vi "Example_Single.vi"() -> ()   [LabVIEW 2015, in "LXM32_Modbus_Serial.lvlib"]
uses:
  LXM32_Modbus_Serial.lvlib
  statistic_indicator.ctl
  register_param.ctl
  <vilib>/Utility/sysdir.llb/System Directory Type.ctl
  <vilib>/Analysis/baseanly.llb/Mean (DBL).vi
  <vilib>/Utility/file.llb/Write Delimited Spreadsheet (string).vi
  <vilib>/Utility/file.llb/Write Delimited Spreadsheet (DBL).vi
  <vilib>/Analysis/NI_AALBase.lvlib
panel:
  in  "Test Name":string="Test"
  in  "Parameter":i32(ring)=3 items=["DC Bus [V]", "Motor Current[Arms]", "Motor Volt [V]", "Actual Torque [%]", "Actual Speed Rot. [rpm]", "Actual Speed Rot. Enc [rpm]", "Actual Velocity", "Actual Velocity of Enc.", "Actual Pos.", "Actual pos. of Enc"]
  in  "LXM Port":refnum<visa-resource-name>
  in  "Stop":bool
  in  "avg":T1={"value"=999.999, "desc"="DC BUS [V]"} caption="Average" {"value" format="%.3f"}
  in  "min":T1={"value"=999.999, "desc"="DC BUS [V]"} caption="Minimum" {"value" format="%.3f"}
  in  "max":T1={"value"=999.999, "desc"="DC BUS [V]"} caption="Maximum" {"value" format="%.3f"}
  in  "nowValue":T1={"value"=999.999, "desc"="DC BUS [V]"} caption="Now Value" {"value" format="%.3f"}
  out "chart":dbl[](graph) caption="Waveform Chart"
  # "LXM32 MODBUS SERIAL"
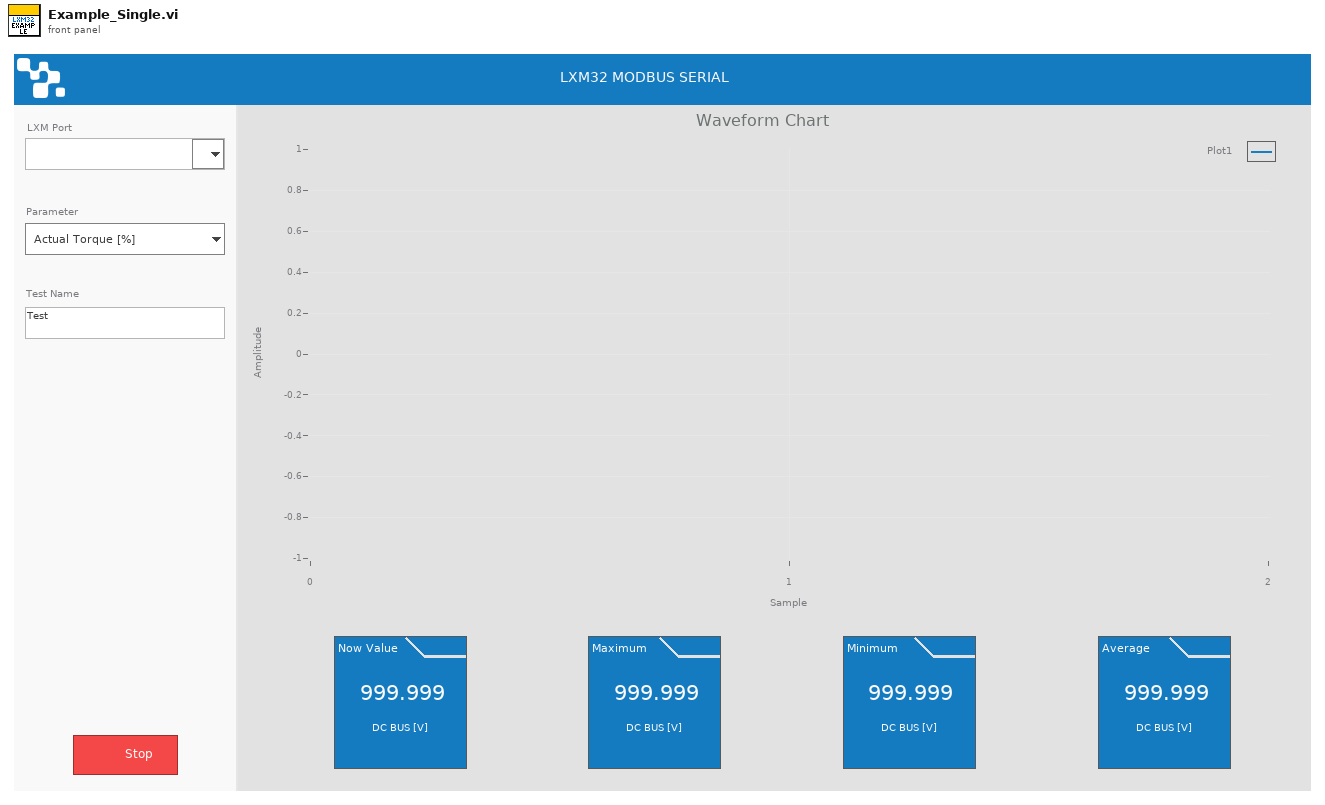
[diagram p1: front panel]
types:
  T1 = typedef "LXM32_Modbus_Serial.lvlib/statistic_indicator.ctl" = cluster{"value":dbl, "desc":string}
  T2 = typedef "System Directory Type.ctl" = i32
  T3 = typedef "LXM32_Modbus_Serial.lvlib/register_param.ctl" = cluster{"name":string, "address":u16, "divisor":dbl}
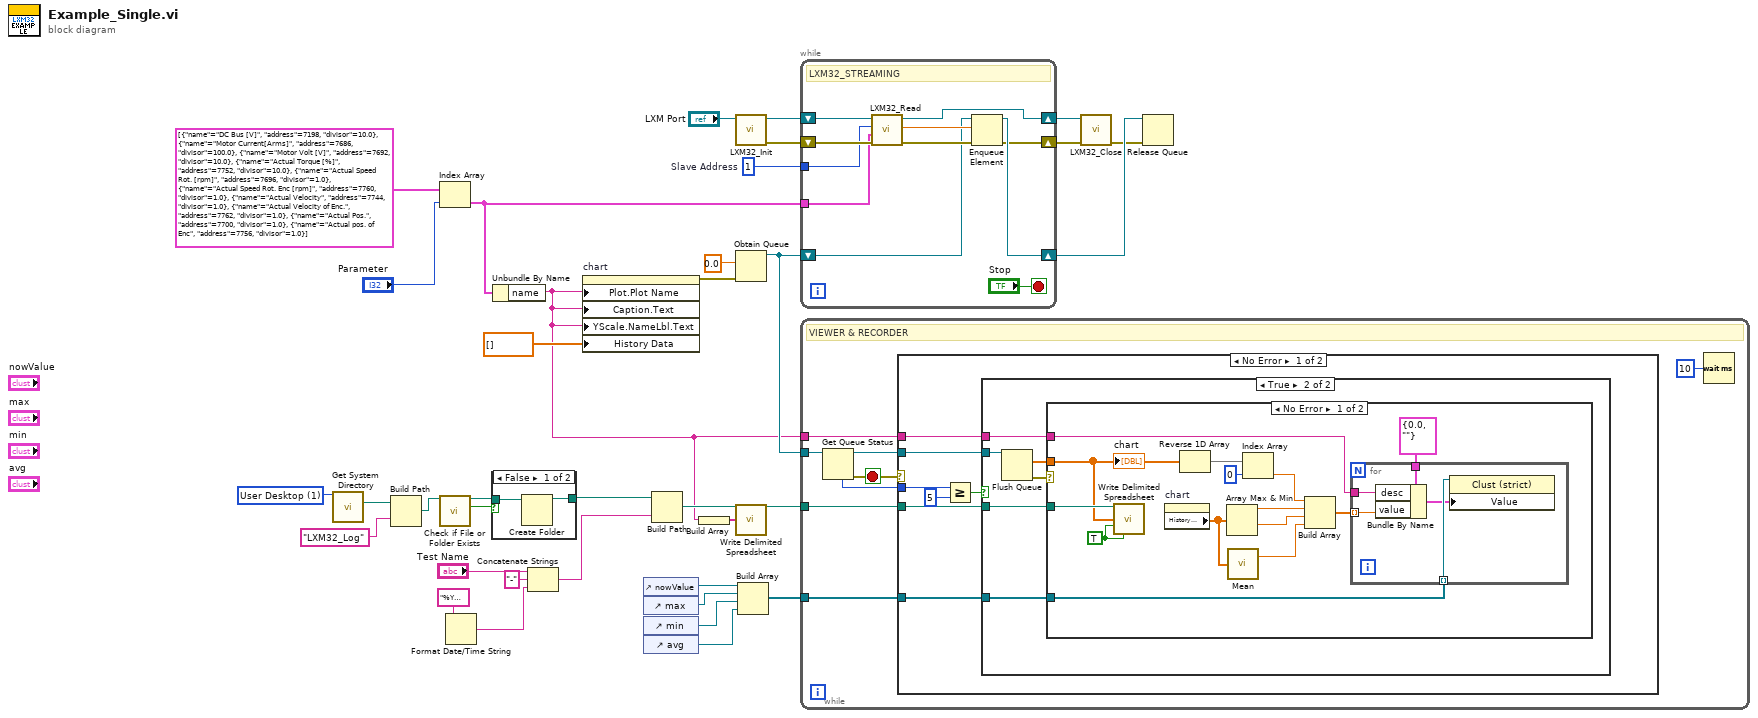
[diagram p0: block diagram]
diagram:
  w30 = T2 1 items=["User Home"=0, "User Desktop"=1, "User Documents"=2, "User Application Data"=3, "User Preferences"=4, "User Temporary"=5, "Public Documents"=6, "Public Application Data"=7, "Public Preferences"=8, "Public Cache"=13, "System Core Libraries"=9, "System Installed Libraries"=10, "Application Files"=11, "Boot Volume Root"=12] ("system directory type")
  w36 = u8 1  # Slave Address
  n1 = call <vilib>:"Get System Directory.vi"("system directory type"=w30) -> ("system directory"=w29:path)  [unwired: 10 in]
  n2 = Build Path(base path=w29, name or relative path="LXM32_Log") -> (appended path=w27:path)
  n3 = Index Array(array=T3[] [{"name"="DC Bus [V]", "address"=7198, "divisor"=10.0}, {"name"="Motor Current[Arms]", "address"=7686, "divisor"=100.0}, {"name"="Motor Volt [V]", "address"=7692, "divisor"=10.0}, {"name"="Actual Torque [%]", "address"=7752, "divisor"=10.0}, {"name"="Actual Speed Rot. [rpm]", "address"=7696, "divisor"=1.0}, {"name"="Actual Speed Rot. Enc [rpm]", "address"=7760, "divisor"=1.0}, {"name"="Actual Velocity", "address"=7744, "divisor"=1.0}, {"name"="Actual Velocity of Enc.", "address"=7762, "divisor"=1.0}, {"name"="Actual Pos.", "address"=7700, "divisor"=1.0}, {"name"="Actual pos. of Enc", "address"=7756, "divisor"=1.0}], index="Parameter") -> (element=w14:T3)
  n4 = call <vilib>:"Check if File or Folder Exists.vi"("path"=w27) -> ("file or folder exists?"=w26:bool, "dup path"=w25:path)  [unwired: 8 in, 1 out]
  n5 = Format Date/Time String(time format string (%c)="%Y%m%d_%H%M%S.txt") -> (date/time string=w2:string)  [unwired: 2 in]
  n6 = case shown="False" w26 {
    tunnel: w25 -> [w38 w39]
    tunnel: [w37 w39] -> w23
    frame False {
      n7 = Create Folder(path (use dialog)=w38) -> (created path=w37:path)  [unwired: 2 in, 2 out]
    }
    frame True {
    }
  }
  n8 = Unbundle By Name(w14) -> ("name"=w5:string)
  n9 = Concatenate Strings("Test Name", "-" ("string"), w2) -> (w1:string)
  n10 = property on="chart" class="WFChart (strict)"("Plot.Plot Name"=w5, "Caption.Text"=w5, "YScale.NameLbl.Text"=w5, "History Data"=dbl[] []) -> (error out=w13:errorcluster)  [unwired: 2 in, 1 out]
  n11 = control-ref of="nowValue"() -> (w11:refnum<vi>)
  n12 = control-ref of="max"() -> (w10:refnum<vi>)
  n13 = control-ref of="min"() -> (w9:refnum<vi>)
  n14 = control-ref of="avg"() -> (w8:refnum<vi>)
  n15 = Build Path(base path=w23, name or relative path=w1) -> (appended path=w22:path)
  n16 = Build Array(w5) -> (w6:string[])
  n17 = call "LXM32_Init.vi"("VISA resource name"="LXM Port") -> ("error out"=w19:errorcluster, "VISA resource name out"=w20:refnum<visa-resource-name>)  [unwired: 9 in]
  n18 = Obtain Queue(element data type=0.0, error in (no error)=w13) -> (queue out=w31:refnum<queue>)  [unwired: 3 in, 2 out]
  n19 = call-poly <vilib>:"Write Delimited Spreadsheet.vi"("file path (dialog if empty)"=w22, "1D data"=w6) -> ("new file path (Not A Path if cancelled)"=w21:path)  [unwired: 12 in, 1 out]
  n20 = Build Array(w11, w10, w9, w8) -> (w7:refnum<vi>[])
  n21 = while {
    shift-right: [w46] -> w35
    shift-left: w20 -> [w50]
    shift-right: [w41] -> w34
    shift-left: w19 -> [w49]
    tunnel: w14 -> [w48]
    tunnel: w36 -> [w47]
    shift-right: [w42] -> w33
    shift-left: w31 -> [w43]
    stop <- "Stop" stop-if-true
    # "LXM32_STREAMING"
    n22 = call "LXM32_Read.vi"("error in"=w49, "register param"=w48, "Slave Address"=w47, "VISA resource name"=w50) -> ("error out"=w45:errorcluster, "value"=w44:dbl, "VISA resource name out"=w46:refnum<visa-resource-name>)  [unwired: 5 in]
    n23 = Enqueue Element(queue=w43, element=w44, error in (no error)=w45) -> (queue out=w42:refnum<queue>, error out=w41:errorcluster)  [unwired: 1 in, 1 out]
  }
  n24 = while {
    tunnel: w31 -> [w55]
    tunnel: w21 -> [w58]
    tunnel: w5 -> [w57]
    tunnel: w7 -> [w56]
    stop <- w54 stop-if-true
    # "VIEWER & RECORDER"
    n25 = Get Queue Status(queue=w55) -> (queue out=w53:refnum<queue>, error out=w54:errorcluster, # elements in queue=w52:i32)  [unwired: 2 in, 5 out]
    n26 = case shown="No Error" w54 {
      tunnel: w58 -> [w65 _]
      tunnel: w57 -> [w64 _]
      tunnel: w56 -> [w63 _]
      tunnel: w53 -> [w59 _]
      tunnel: w52 -> [w62 _]
      frame No Error {
        n27 = Greater Or Equal?(x=w62, y=5) -> (x >= y?=w60:bool)
        n28 = case shown="True" w60 {
          tunnel: w65 -> [_ w71]
          tunnel: w64 -> [_ w70]
          tunnel: w63 -> [_ w69]
          tunnel: w59 -> [_ w68]
          frame False {
          }
          frame True {
            n29 = Flush Queue(queue=w68) -> (remaining elements=w66:dbl[], error out=w67:errorcluster)  [unwired: 1 in, 1 out]
            n30 = case shown="No Error" w67 {
              tunnel: w71 -> [w85 _]
              tunnel: w70 -> [w78 _]
              tunnel: w69 -> [w77 _]
              tunnel: w66 -> [w73 _]
              frame No Error {
                w72 = TRUE ("append to file? (F)")
                n31 = call-poly <vilib>:"Write Delimited Spreadsheet.vi"("file path (dialog if empty)"=w85, "1D data"=w73, "append to file? (F)"=w72, "transpose? (F)"=w72) -> ()  [unwired: 10 in, 2 out]
                n32 = property on="chart" class="WFChart (strict)"() -> ("History Data"=w79:dbl[])  [unwired: 2 in, 2 out]
                n33 = Reverse 1D Array(array=w73) -> (reversed array=w76:dbl[])
                n34 = Array Max & Min(array=w79) -> (max value=w80:dbl, min value=w81:dbl)  [unwired: 2 out]
                n35 = call-poly <vilib>:"Mean.vi"("X"=w79) -> ("mean"=w82:dbl)  [unwired: 1 out]
                n36 = Index Array(array=w76, index=0) -> (element=w74:dbl)
                n37 = Build Array(w74, w80, w81, w82) -> (w83:dbl[])
                n38 = for {
                  tunnel: w83 -> [w90] mode=indexing
                  tunnel: T1 {"value"=0.0, "desc"=""} ("nowValue") -> [w89]
                  tunnel: w78 -> [w88]
                  tunnel: w77 -> [w87] mode=indexing
                  n39 = Bundle By Name(cluster=w89, "desc"=w88, "value"=w90) -> (w86:T1)
                  n40 = property class="Clust (strict)"(reference=w87, "Value"=w86) -> ()  [unwired: 1 in, 2 out]
                }
                "chart" <- w73
              }
              frame Error {
              }
            }
          }
        }
      }
      frame Error {
      }
    }
    n41 = Wait (ms)(milliseconds to wait=u32 10) -> ()  [unwired: 1 out]
  }
  n42 = call "LXM32_Close.vi"("error in"=w34, "VISA resource name"=w35) -> ("error out"=w32:errorcluster)  [unwired: 9 in]
  n43 = Release Queue(queue=w33, error in (no error)=w32) -> ()  [unwired: 1 in, 3 out]
